vi "Build Light Map.vi"(8 "error in":errorcluster, 9 "Light Data":string[](array[string]), 10 "Light IDs":i32[](array[numeric])) -> (0 "error out":errorcluster, 2 "Light Map":map{i32, T1}(c390))   [LabVIEW 2020, in "LMH-Hue.lvlib"]
uses:
  LMH-Hue.lvlib
  Type Defs/Light Data.ctl
  <vilib>/JDP Science/JSONtext/String Subset.vi
  <vilib>/JDP Science/JSONtext/support/Quote and Escape JSON string.vi
  <vilib>/JDP Science/JSONtext/support/quote and escape json string 2.vi
  <vilib>/JDP Science/JSONtext/Parsing/Parse Full Path or Item Name.vi
  <vilib>/JDP Science/JSONtext/Offset/Find Item Locations by Path.vi
  <vilib>/JDP Science/JSONtext/Offset/Find Object Item Locations by Names.vi
  <vilib>/JDP Science/JSONtext/JSONtext.lvlib
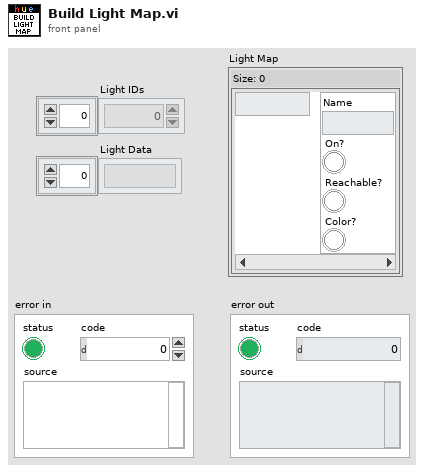
[diagram p1: front panel]
types:
  T1 = typedef "LMH-Hue.lvlib/Light Data.ctl" = cluster{"Name":string, "On?":bool, "Reachable?":bool, "Color?":bool}
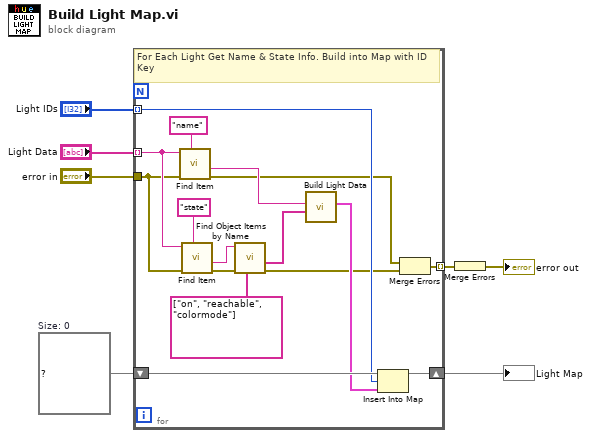
[diagram p0: block diagram]
diagram:
  w5 = map{i32, T1} {}  # Size: 0
  n1 = for {
    tunnel: "Light Data" -> [w21] mode=indexing
    tunnel: "Light IDs" -> [w16] mode=indexing
    shift-right: [w17] -> w1
    shift-left: w5 -> [w18]
    tunnel: "error in" -> [w11]
    tunnel: [w8] -> w3 mode=indexing
    # "For Each Light Get Name & State Info. Build into Map with ID Key"
    n2 = call <vilib>:"Find Item.vi"("$Path or Item Name"="name", "error in (no error)"=w11, "JSON"=w21) -> ("error out"=w10:errorcluster, "<JSON>"=w13:string)  [unwired: 5 in, 2 out]
    n3 = call <vilib>:"Find Item.vi"("$Path or Item Name"="state", "error in (no error)"=w11, "JSON"=w21) -> ("error out"=w12:errorcluster, "<JSON>"=w20:string)  [unwired: 5 in, 2 out]
    n4 = call <vilib>:"Find Object Items by Name.vi"("Item Names"=string[] ["on", "reachable", "colormode"], "error in (no error)"=w12, "JSON"=w20) -> ("error out"=w9:errorcluster, "<JSON>"=w15:string[])  [unwired: 6 in, 1 out]
    n5 = call "Build Light Data.vi"("Light State Info"=w15, "Light Name"=w13) -> ("Light Data"=w14:T1)  [unwired: 9 in]
    n6 = Insert Into Map(map in=w18, key=w16, value=w14) -> (map out=w17:map{i32, T1})  [unwired: 2 out]
    n7 = Merge Errors(w10, w9) -> (w8:errorcluster)
  }
  "Light Map" <- w1
  n8 = Merge Errors(w3) -> (→"error out":errorcluster)
